vi "write vi connector panes to files.vi"() -> ()   [LabVIEW 2024]
panel:
  out "error out":errorcluster
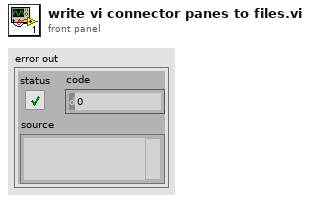
[diagram p1: front panel]
types:
  T1 = enum16{"open", "replace", "create", "open or create", "replace or create", "replace or create with confirmation"}
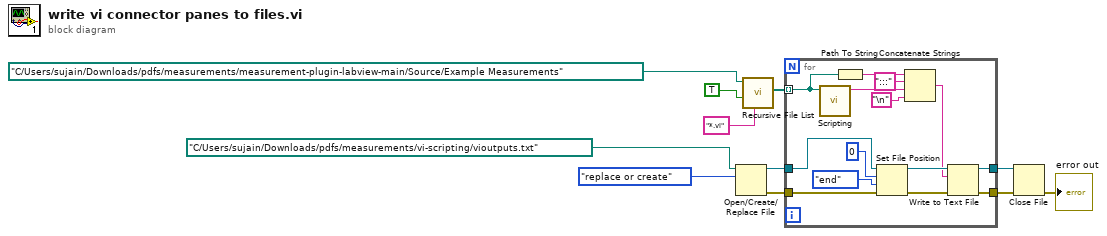
[diagram p0: block diagram]
diagram:
  n1 = Open/Create/Replace File(file path (use dialog)=path "C:/Users/sujain/Downloads/pdfs/measurements/vi-scripting/vioutputs.txt", operation (0:open)=T1."replace or create") -> (refnum out=w5:refnum<file>, error out=w2:errorcluster)  [unwired: 4 in, 1 out]
  n2 = call <vilib>:"Recursive File List.vi"("pattern"="*.vi", "Continue Recursing on Error? (F)"=TRUE, "Folder Path"=path "C:/Users/sujain/Downloads/pdfs/measurements/measurement-plugin-labview-main/Source/Example Measurements") -> ("All Files in Dir"=w8:path[])  [unwired: 4 in, 4 out]
  n3 = for {
    tunnel: w8 -> [w14] mode=indexing
    tunnel: w5 -> [w25]
    tunnel: [w22] -> w4
    tunnel: [w21] -> w3
    tunnel: w2 -> [w15]
    n4 = call "Scripting.vi"("vi path"=w14) -> ("String"=w19:string)  [unwired: 10 in]
    n5 = Path To String(path=w14) -> (string=w13:string)
    n6 = Set File Position(offset (in bytes) (0)=i64 0, refnum=w25, from (0:start)=enum16{"start", "end", "current"}."end", error in=w15) -> (refnum out=w20:refnum<file>, error out=w16:errorcluster)
    n7 = Concatenate Strings(w13, ":::" ("string"), w19, "\n") -> (w17:string)
    n8 = Write to Text File(file (use dialog)=w20, text=w17, error in=w16) -> (refnum out=w21:refnum<file>, error out=w22:errorcluster)  [unwired: 1 in, 1 out]
  }
  n9 = Close File(refnum=w3, error in=w4) -> (error out=→"error out":errorcluster)  [unwired: 1 out]
